vi "PIC_Init_Serial_Term.vi"(8 "error in (no error)":errorcluster, 10 "Interface protocol":T1(ring), 11 "VISA resource name":refnum<visa-resource-name>) -> (0 "error out":errorcluster, 3 "VISA resource name Out":refnum<visa-resource-name>)   [LabVIEW 2017]
uses:
  <vilib>/Instr/_visa.llb/Select Event Type.ctl
  <vilib>/Instr/_visa.llb/VISA Configure Serial Port (Instr).vi
panel:
  out "read buffer":string
  out "FW Version":string
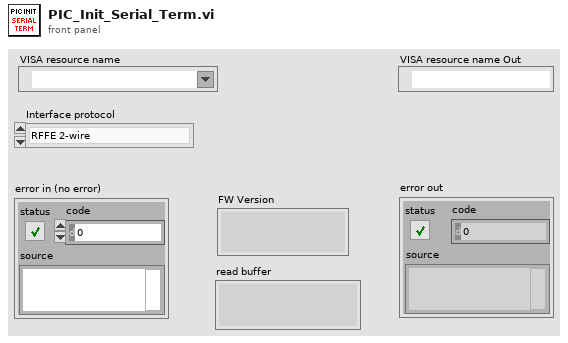
[diagram p1: front panel]
types:
  T1 = enum16{"RFFE 2-wire", "WiSPI 3-wire spi_sel", "WiSPI 4-wire spi_sel", "ifxSPI 3-wire spi_sel", "WiSPI 3-wire dev add spi_sel"}
  T2 = typedef "Select Event Type.ctl" = u32
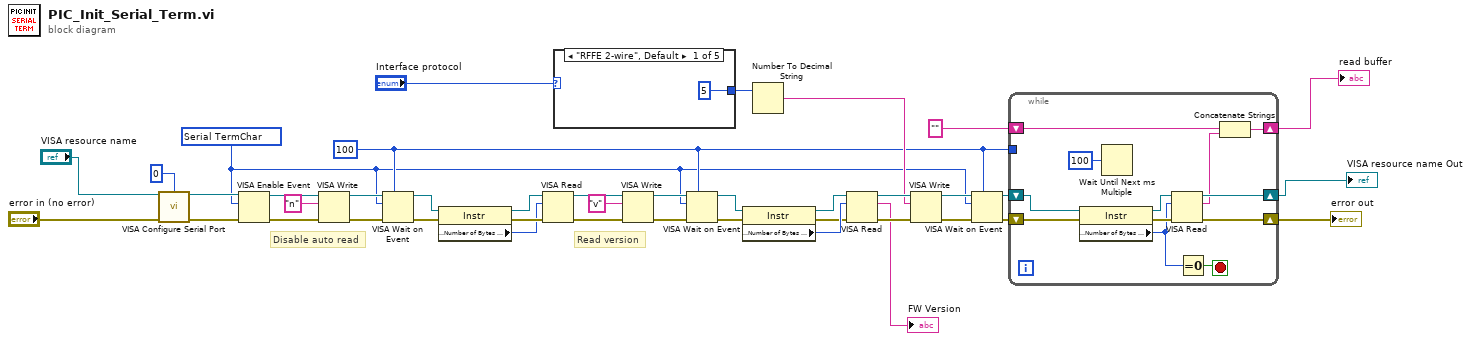
[diagram p0: block diagram]
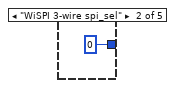
[diagram p2: hidden frame]
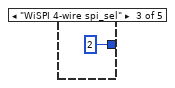
[diagram p3: hidden frame]
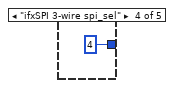
[diagram p4: hidden frame]
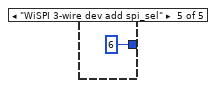
[diagram p5: hidden frame]
diagram:
  w5 = u32 100 ("timeout (0)")
  w4 = T2 1073684516 items=["Service Request"=1073684491, "Trigger"=3221168138, "Clear"=1073684493, "VXI Signal"=1073684512, "VXI/VME Interrupt"=3221168161, "VXI/VME Sysfail"=1073684509, "VXI/VME Sysreset"=1073684510, "GPIB CIC"=1073684498, "GPIB Talk"=1073684499, "GPIB Listen"=1073684500, "PXI Interrupt"=1073684514, "Serial Break"=1073684515, "Serial TermChar"=1073684516, "Serial CTS"=1073684521, "Serial DSR"=1073684522, "Serial DCD"=1073684524, "Serial RI"=1073684526, "Serial Character"=1073684533, "USB Interrupt"=1073684535, "All Enabled"=1073709055] ("Event Type")
  # "Read version"
  # "Disable auto read"
  n1 = call-poly "VISA Configure Serial Port"("VISA resource name"="VISA resource name", "termination char\n(0xA = '\\n' = LF)"=u8 0 ("termination char\n(0xA = '\\n' = LF)"), "error in (no error)"="error in (no error)") -> ("VISA resource name out"=w39:refnum<visa-resource-name>, "error out"=w40:errorcluster)  [unwired: 11 in]
  n2 = VISA Enable Event(8:w40, 10:w4, 11:w39) -> (0:w38:errorcluster, 3:w37:refnum<visa-resource-name>)  [unwired: 1 in]
  n3 = VISA Write(VISA resource name=w37, write buffer="n", error in (no error)=w38) -> (VISA resource name out=w34:refnum<visa-resource-name>, error out=w35:errorcluster)  [unwired: 1 out]
  n4 = VISA Wait on Event(7:w5, 8:w35, 10:w4, 11:w34) -> (0:w32:errorcluster, 3:w33:refnum<visa-resource-name>)  [unwired: 1 in, 2 out]
  n5 = property class="Instr"(reference=w33, error in=w32) -> (reference out=w29:refnum<visa-resource-name>, error out=w31:errorcluster, "Serial Settings:Number of Bytes at Serial Port"=w30:u32)
  n6 = VISA Read(VISA resource name=w29, byte count=w30, error in (no error)=w31) -> (VISA resource name out=w20:refnum<visa-resource-name>, error out=w19:errorcluster)  [unwired: 2 out]
  n7 = case shown="\"RFFE 2-wire\", Default" "Interface protocol" {
    tunnel: [5 0 2 4 6] -> w16
    frame "RFFE 2-wire", Default {
    }
    frame "WiSPI 3-wire spi_sel" {
    }
    frame "WiSPI 4-wire spi_sel" {
    }
    frame "ifxSPI 3-wire spi_sel" {
    }
    frame "WiSPI 3-wire dev add spi_sel" {
    }
  }
  n8 = VISA Write(VISA resource name=w20, write buffer="v", error in (no error)=w19) -> (VISA resource name out=w23:refnum<visa-resource-name>, error out=w22:errorcluster)  [unwired: 1 out]
  n9 = VISA Wait on Event(7:w5, 8:w22, 10:w4, 11:w23) -> (0:w25:errorcluster, 3:w24:refnum<visa-resource-name>)  [unwired: 1 in, 2 out]
  n10 = property class="Instr"(reference=w24, error in=w25) -> (reference out=w28:refnum<visa-resource-name>, error out=w26:errorcluster, "Serial Settings:Number of Bytes at Serial Port"=w27:u32)
  n11 = Number To Decimal String(number=w16) -> (decimal integer string=w15:string)  [unwired: 1 in]
  n12 = VISA Read(VISA resource name=w28, byte count=w27, error in (no error)=w26) -> (VISA resource name out=w17:refnum<visa-resource-name>, read buffer=→"FW Version":string, error out=w18:errorcluster)  [unwired: 1 out]
  n13 = VISA Write(VISA resource name=w17, write buffer=w15, error in (no error)=w18) -> (VISA resource name out=w6:refnum<visa-resource-name>, error out=w7:errorcluster)  [unwired: 1 out]
  n14 = VISA Wait on Event(7:w5, 8:w7, 10:w4, 11:w6) -> (0:w2:errorcluster, 3:w3:refnum<visa-resource-name>)  [unwired: 1 in, 2 out]
  n15 = while {
    tunnel: w5 -> [_]
    shift-right: [w55] -> w10
    shift-left: w2 -> [w48]
    shift-right: [w56] -> w1
    shift-left: w3 -> [w47]
    shift-right: [w54] -> w12
    shift-left: "" -> [w52]
    stop <- w50 stop-if-true
    n16 = property class="Instr"(reference=w47, error in=w48) -> (reference out=w57:refnum<visa-resource-name>, error out=w58:errorcluster, "Serial Settings:Number of Bytes at Serial Port"=w49:u32)
    n17 = Wait Until Next ms Multiple(millisecond multiple=u32 100) -> ()  [unwired: 1 out]
    n18 = VISA Read(VISA resource name=w57, byte count=w49, error in (no error)=w58) -> (VISA resource name out=w56:refnum<visa-resource-name>, read buffer=w53:string, error out=w55:errorcluster)  [unwired: 1 out]
    n19 = Equal To 0?(x=w49) -> (x = 0?=w50:bool)
    n20 = Concatenate Strings(w52, w53) -> (w54:string)
  }
  "read buffer" <- w12
  "VISA resource name Out" <- w1
  "error out" <- w10
